vi "SRV_PM_Is Packet Complete.vi"(0 "Packet Data":u8[](array[numeric]) format="%.0x", 11 "error in (no error)":errorcluster) -> (4 "Packet Data dup":u8[](array[numeric]) format="%.0x", 8 "Packet Complete?":bool, 10 "Total Packet Length":u16, 15 "error out":errorcluster)   [LabVIEW 2014]
panel:
  out "Data Field Length":u16
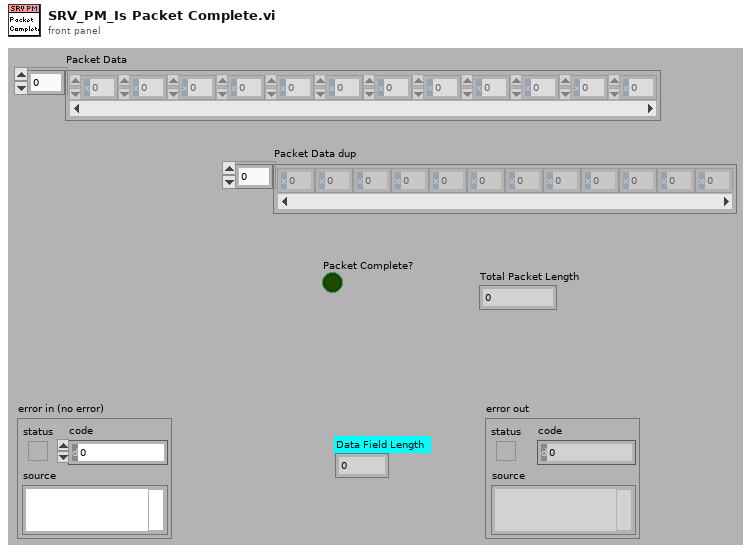
[diagram p1: front panel]
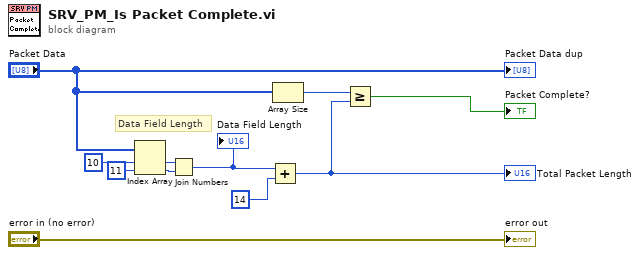
[diagram p0: block diagram]
diagram:
  # "Data Field Length"
  n1 = Index Array(array="Packet Data", index #1=10 ("index"), index #2=11 ("index")) -> (element #1=w6:u8, element #2=w5:u8)
  n2 = Join Numbers(hi=w6, lo=w5) -> ((hi.lo)=w1:u16)
  "Data Field Length" <- w1
  n3 = Add(x=w1, y=u16 14) -> (x+y=w7:u16)
  "Total Packet Length" <- w7
  n4 = Array Size(array="Packet Data") -> (size(s)=w8:i32)
  n5 = Greater Or Equal?(x=w8, y=w7) -> (x >= y?=→"Packet Complete?":bool)
  "Packet Data dup" <- "Packet Data"
  "error out" <- "error in (no error)"
